vi "WriteSLMPAttern.vi"(8 "Holo Array":T1[](array[typedef]), 11 "General settings":T4) -> (3 "Display Array":u8[][](array[numeric]))   [LabVIEW 2018]
uses:
  Controls/General Setting.ctl
  Controls/Buttons/Running Button.ctl
  Controls/Holo Setting.ctl
  Controls/Zernike Polynominals.ctl
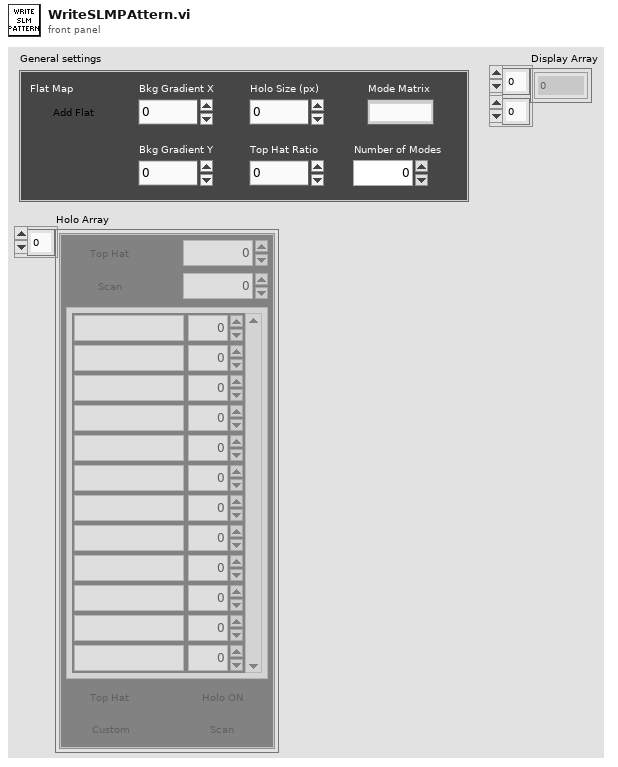
[diagram p1: front panel]
types:
  T1 = typedef "Holo Setting.ctl" = cluster{"Holo On":T2, "Scan":T2, "X":i16, "Y":i16, "Zernike Polynominals":T3, "Top Hat":T2, "Vortex":T2, "Clockwise":T2, "Custom":T2}
  T2 = typedef "Running Button.ctl" = bool
  T3 = typedef "Zernike Polynominals.ctl" = cluster{"Aberration Name":string, "Numeric":dbl}[]
  T4 = typedef "General Setting.ctl" = cluster{"Flat Map":T2, "Bkg Gradient X":dbl, "Bkg Gradient Y":dbl, "Holo Size (px)":i32, "Top Hat Ratio":dbl, "Number of Modes":i8, "Mode Matrix":u16}
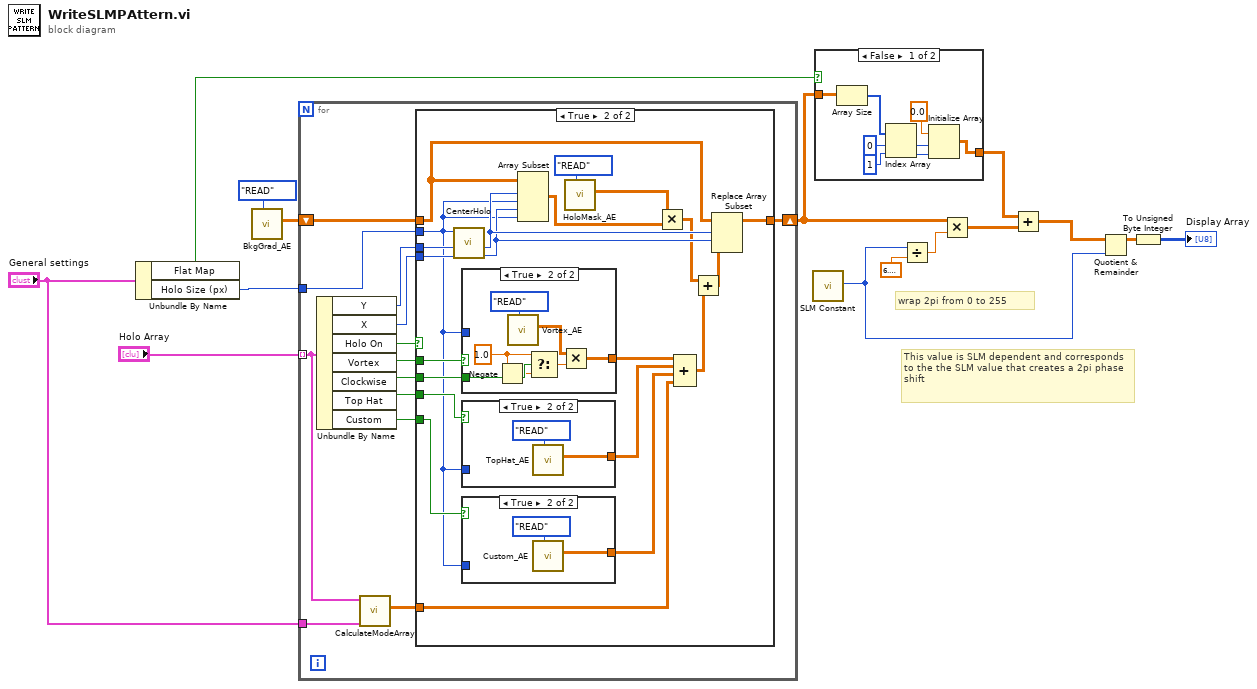
[diagram p0: block diagram]
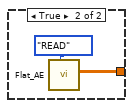
[diagram p2: hidden frame]
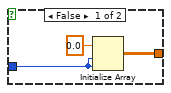
[diagram p4: hidden frame]
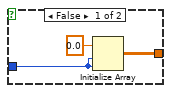
[diagram p5: hidden frame]
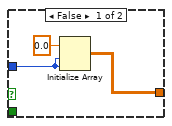
[diagram p6: hidden frame]
diagram:
  # "This value is SLM dependent and corresponds to the the SLM value that creates a 2pi phase shift"
  # "wrap 2pi from 0 to 255"
  n1 = Unbundle By Name("General settings") -> ("Flat Map"=w12:T2, "Holo Size (px)"=w5:i32)
  n2 = call "BkgGrad_AE.vi"("Action"=enum16{"READ", "WRITE"}."READ") -> ("BkgGrad Out"=w9:dbl[][])  [unwired: 10 in]
  n3 = for {
    tunnel: "Holo Array" -> [w18] mode=indexing
    tunnel: w5 -> [w24]
    shift-right: [w20] -> w6
    shift-left: w9 -> [w21]
    tunnel: "General settings" -> [w17]
    n4 = Unbundle By Name(w18) -> ("Y"=w23:i16, "X"=w22:i16, "Holo On"=w25:T2, "Vortex"=w28:T2, "Clockwise"=w27:T2, "Top Hat"=w26:T2, "Custom"=w16:T2)
    n5 = call "CalculateModeArray.vi"("General settings"=w17, "Holo Settings"=w18) -> ("ModeArray"=w19:dbl[][])  [unwired: 9 in]
    n6 = case shown="True" w25 {
      tunnel: w28 -> [_ w46]
      tunnel: w27 -> [_ w50]
      tunnel: w21 -> [w29 w42]
      tunnel: w26 -> [_ w45]
      tunnel: w24 -> [_ w32]
      tunnel: w23 -> [_ w49]
      tunnel: w22 -> [_ w48]
      tunnel: [w29 w43] -> w20
      tunnel: w19 -> [_ w31]
      tunnel: w16 -> [_ w33]
      frame False {
      }
      frame True {
        n7 = call "CenterHolo.vi"("X"=w48, "Y"=w49, "Holo Size"=w32) -> ("X centered"=w40:i32, "Y centered"=w41:i32)  [unwired: 7 in]
        n8 = case shown="True" w46 {
          tunnel: w50 -> [_ w70]
          tunnel: [w62 w64] -> w39
          tunnel: w32 -> [w61 _]
          frame False {
            n9 = Initialize Array(0.0 ("element"), w61, w61) -> (w62:dbl[][])
          }
          frame True {
            w69 = 1.0 ("t")
            n10 = Negate(x=w69) -> (-x=w68:dbl)
            n11 = call "Vortex_AE.vi"("Action"=enum16{"READ", "WRITE"}."READ") -> ("Vortex Out"=w66:dbl[][])  [unwired: 10 in]
            n12 = Select(t=w69, s=w70, f=w68) -> (s? t:f=w65:dbl)
            n13 = Multiply(x=w66, y=w65) -> (x*y=w64:dbl[][])
          }
        }
        n14 = case shown="True" w45 {
          tunnel: [w57 w59] -> w44
          tunnel: w32 -> [w56 _]
          frame False {
            n15 = Initialize Array(0.0 ("element"), w56, w56) -> (w57:dbl[][])
          }
          frame True {
            n16 = call "TopHat_AE.vi"("Action"=enum16{"READ", "WRITE"}."READ") -> ("TopHat Out"=w59:dbl[][])  [unwired: 10 in]
          }
        }
        n17 = case shown="True" w33 {
          tunnel: [w52 w54] -> w30
          tunnel: w32 -> [w51 _]
          frame False {
            n18 = Initialize Array(0.0 ("element"), w51, w51) -> (w52:dbl[][])
          }
          frame True {
            n19 = call "Custom_AE.vi"("Action"=enum16{"READ", "WRITE"}."READ") -> ("Custom Out"=w54:dbl[][])  [unwired: 10 in]
          }
        }
        n20 = Array Subset(array=w42, index (row)=w41, length (row)=w32, index (col)=w40, length (col)=w32) -> (w34:dbl[][])
        n21 = call "HoloMask_AE.vi"("Action"=enum16{"READ", "WRITE"}."READ") -> ("HoloMask Out"=w35:dbl[][])  [unwired: 10 in]
        n22 = Multiply(x=w35, y=w34) -> (x*y=w38:dbl[][])
        n23 = Compound Arithmetic op=ADD(w39, w44, w30, w31) -> (w36:dbl[][])
        n24 = Add(x=w38, y=w36) -> (x+y=w37:dbl[][])
        n25 = Replace Array Subset(array=w42, new element=w37, index (row)=w41, index (col)=w40) -> (w43:dbl[][])
      }
    }
  }
  n26 = call "SLM Constant.vi"() -> ("Gray Level Corresponding to 2Pi"=w4:i32)  [unwired: 10 in, 9 out]
  n27 = case shown="False" w12 {
    tunnel: [w71 w79] -> w13
    tunnel: w6 -> [w72 _]
    frame False {
      n28 = Array Size(array=w72) -> (size(s)=w74:i32[])
      n29 = Index Array(array=w74, index #1=0 ("index"), index #2=1 ("index")) -> (element #1=w76:i32, element #2=w77:i32)
      n30 = Initialize Array(0.0 ("element"), w76, w77) -> (w71:dbl[][])
    }
    frame True {
      n31 = call "Flat_AE.vi"("Action"=enum16{"READ", "WRITE"}."READ") -> ("Flat Out"=w79:dbl[][])  [unwired: 10 in]
    }
  }
  n32 = Divide(x=w4, y=6.283185307179586) -> (x/y=w10:dbl)
  n33 = Multiply(x=w6, y=w10) -> (x*y=w1:dbl[][])
  n34 = Add(x=w13, y=w1) -> (x+y=w3:dbl[][])
  n35 = Quotient & Remainder(x=w3, y=w4) -> (x-y*floor(x/y)=w14:dbl[][])  [unwired: 1 out]
  n36 = To Unsigned Byte Integer(number=w14) -> (unsigned 8bit integer=→"Display Array":u8[][])
